vi "Add Frame.vi"(8 "error in (no error)":errorcluster, 11 "Node Ptr":u64 format="%.0x") -> (0 "error out":errorcluster)   [LabVIEW 2015, in "Diagnostics Addon System Explorer.lvlib"]
uses:
  Diagnostics Addon System Explorer.lvlib
  Shared/Types/MessageType Selector.ctl
  Shared/Types/Frame Parameters.ctl
  Shared/Types/Signal Parameters.ctl
  Shared/SubVIs/GUID Lookup.vi
  <vilib>/NI Veristand/Custom Device API/Custom Device API.lvlib
  Shared/Diagnostics Addon Shared.lvlib
  <vilib>/NI Veristand/Custom Device Tools/Custom Device Utility Library/Custom Device Utility Library.lvlib
panel:
  in  "Tag":string
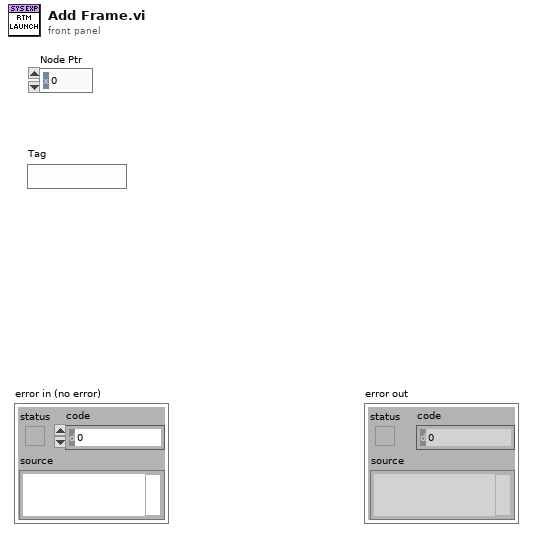
[diagram p1: front panel]
types:
  T1 = typedef "Custom Device API.lvlib/Custom Device Item Ref.ctl" = u64
  T2 = typedef "Custom Device API.lvlib/Custom Device Item Info.ctl" = cluster{"Name":string, "Is Channel":bool, "GUID":string, "Is Waveform":bool}
  T3 = typedef "Diagnostics Addon Shared.lvlib/MessageType Selector.ctl" = enum16{"DID", "PID", "CPID", "Write Memory", "Read Memory", "DTC Control", "IO Cmd", "IO Resp", "Routine Start Cmd", "Routine Start Resp", "Routine Status Cmd", "Routine Status Resp", "Routine Stop Cmd", "Routine Stop Resp"}
  T4 = typedef "Diagnostics Addon Shared.lvlib/Signal Parameters.ctl" = cluster{"Start Bit":u8, "Length":u8, "Scaling Factor":dbl, "Scaling Offset":dbl, "Minimum":dbl, "Maximum":dbl, "Data Type":u32, "Byte Order":u32, "Default Value":dbl, "Name":string, "Units":string, "Description":string}
  T5 = typedef "Diagnostics Addon Shared.lvlib/Frame Parameters.ctl" = cluster{"Name":string, "Description":string, "ID":u32, "Type":T3, "Signals":T4[]}
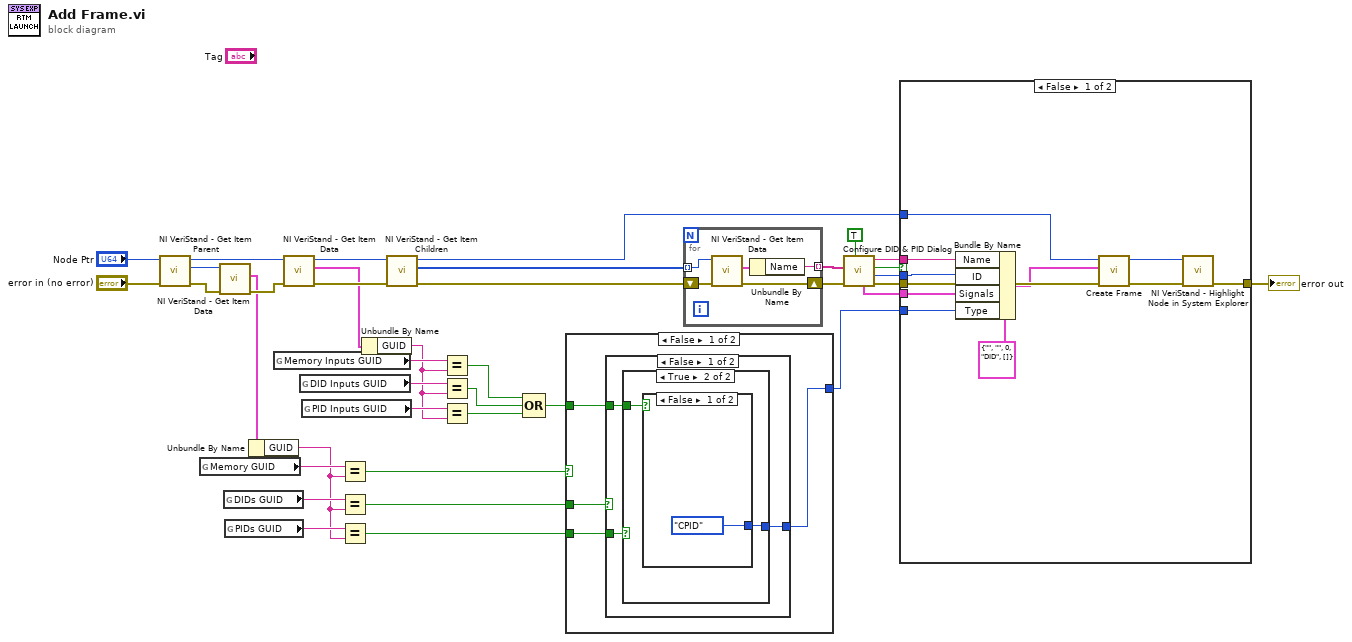
[diagram p0: block diagram]
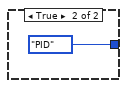
[diagram p3: hidden frame]
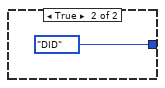
[diagram p4: hidden frame]
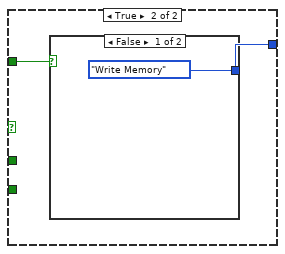
[diagram p5: hidden frame]
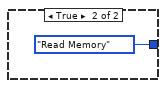
[diagram p6: hidden frame]
diagram:
  n1 = call <vilib>:"NI VeriStand - Get Item Parent.vi"("error in (no error)"="error in (no error)", "Item Ref in"="Node Ptr") -> ("error out"=w12:errorcluster, "Parent Ref"=w13:T1, "Item Ref out"=w14:T1)  [unwired: 6 in, 1 out]
  n2 = global read "GUID Lookup.vi" "Memory GUID"() -> (w9:string)
  n3 = call <vilib>:"NI VeriStand - Get Item Data.vi"("error in (no error)"=w12, "Item Ref in"=w13) -> ("error out"=w11:errorcluster, "Item Info"=w10:T2)  [unwired: 6 in, 2 out]
  n4 = global read "GUID Lookup.vi" "DIDs GUID"() -> (w8:string)
  n5 = global read "GUID Lookup.vi" "PIDs GUID"() -> (w7:string)
  n6 = Unbundle By Name(w10) -> ("GUID"=w6:string)
  n7 = global read "GUID Lookup.vi" "Memory Inputs GUID"() -> (w21:string)
  n8 = call <vilib>:"NI VeriStand - Get Item Data.vi"("error in (no error)"=w11, "Item Ref in"=w14) -> ("error out"=w29:errorcluster, "Item Info"=w27:T2, "Item Ref out"=w28:T1)  [unwired: 6 in, 1 out]
  n9 = global read "GUID Lookup.vi" "DID Inputs GUID"() -> (w22:string)
  n10 = global read "GUID Lookup.vi" "PID Inputs GUID"() -> (w26:string)
  n11 = Equal?(x=w9, y=w6) -> (x = y?=w3:bool)
  n12 = Equal?(x=w8, y=w6) -> (x = y?=w4:bool)
  n13 = Equal?(x=w7, y=w6) -> (x = y?=w5:bool)
  n14 = Unbundle By Name(w27) -> ("GUID"=w20:string)
  n15 = call <vilib>:"NI VeriStand - Get Item Children.vi"("error in (no error)"=w29, "Item Ref in"=w28) -> ("error out"=w38:errorcluster, "Child Refs"=w31:T1[], "Item Ref out"=w30:T1)  [unwired: 6 in, 1 out]
  n16 = Equal?(x=w21, y=w20) -> (x = y?=w17:bool)
  n17 = Equal?(x=w22, y=w20) -> (x = y?=w18:bool)
  n18 = Equal?(x=w26, y=w20) -> (x = y?=w19:bool)
  n19 = Compound Arithmetic op=OR(w17, w18, w19) -> (w2:bool)
  n20 = case shown="False" w3 {
    tunnel: w5 -> [w42 _]
    tunnel: w4 -> [w41 _]
    tunnel: [w40 w52] -> w1
    tunnel: w2 -> [w39 w51]
    frame False {
      n21 = case shown="False" w41 {
        tunnel: w42 -> [w45 _]
        tunnel: [w44 MessageType_Selector."DID" ("Type")] -> w40
        tunnel: w39 -> [w43 _]
        frame False {
          n22 = case shown="True" w45 {
            tunnel: [_ w47] -> w44
            tunnel: w43 -> [_ w46]
            frame False {
            }
            frame True {
              n23 = case shown="False" w46 {
                tunnel: [MessageType_Selector."CPID" ("Type") MessageType_Selector."PID" ("Type")] -> w47
                frame False {
                }
                frame True {
                }
              }
            }
          }
        }
        frame True {
        }
      }
    }
    frame True {
      n24 = case shown="False" w51 {
        tunnel: [MessageType_Selector."Write Memory" ("Type") MessageType_Selector."Read Memory" ("Type")] -> w52
        frame False {
        }
        frame True {
        }
      }
    }
  }
  n25 = for {
    tunnel: [w57] -> w37 mode=indexing
    shift-right: [w56] -> w36
    shift-left: w38 -> [w58]
    tunnel: w31 -> [w55] mode=indexing
    n26 = call <vilib>:"NI VeriStand - Get Item Data.vi"("error in (no error)"=w58, "Item Ref in"=w55) -> ("error out"=w56:errorcluster, "Item Info"=w59:T2)  [unwired: 8 out]
    n27 = Unbundle By Name(w59) -> ("Name"=w57:string)
  }
  n28 = call "Configure DID & PID Dialog.vi"("Show Name&ID"=TRUE, "error in (no error)"=w36, "Existing PIDs"=w37) -> ("error out"=w34:errorcluster, "ID out"=w25:u16, "Cancel PID?"=w35:bool, "Name out"=w33:string, "Signals out"=w24:T4[])  [unwired: 4 in]
  n29 = case shown="False" w35 {
    tunnel: w34 -> [w70 w71]
    tunnel: w30 -> [w69 _]
    tunnel: w33 -> [w67 _]
    tunnel: [w68 w71] -> w32
    tunnel: w25 -> [w66 _]
    tunnel: w24 -> [w65 _]
    tunnel: w1 -> [w60 _]
    frame False {
      n30 = Bundle By Name(cluster=T5 {"Name"="", "Description"="", "ID"=0, "Type"=enum."DID", "Signals"=[]} ("DIDPID"), "Name"=w67, "ID"=w66, "Signals"=w65, "Type"=w60) -> (w61:T5)
      n31 = call "Create Frame.vi"("error in (no error)"=w70, "Frame"=w61, "Section Ptr"=w69) -> ("error out"=w63:errorcluster, "Parent Ref out"=w64:T1)  [unwired: 7 in]
      n32 = call <vilib>:"NI VeriStand - Highlight Node in System Explorer.vi"("error in (no error)"=w63, "Item Ref in"=w64) -> ("error out"=w68:errorcluster)  [unwired: 8 in, 1 out]
    }
    frame True {
    }
  }
  "error out" <- w32
